vi "Create Zero Plane.vi"(7 "3D Waterfall Property":T1={"General Property"={"Plot Name"="", "Coordinate System"=enum."Cartesian", "Opacity"=0.0}, "Projection Property"={"Draw XY"=FALSE, "Draw YZ"=FALSE, "Draw XZ"=FALSE}, "Plot Property"={"Line Style"=enum."None", "Line Width"=0.0, "Color Ramp Cluster"={"Color Ramp Style"=enum."None", "Color Ramp Array"=[16711934, 393471, 57855, 4390754, 16449346, 16744722, 16711680], "Color Ramp Index"=[45, 91, 133, 175, 219, 255], "Interpolate?"=FALSE, "Logarithm?"=FALSE}, "Antialiasing"=FALSE}, "Waterfall Property"={"Waterfall Mode"=enum."Lines"}}, 8 "error in (no error)":errorcluster, 9 "Actual Transform In":T7, 10 "Plot Representation In":T4, 11 "Plot Object In":refnum<vi>) -> (0 "error out":errorcluster, 1 "Actual Transform Out":T7, 2 "Plot Representation Out":T4, 3 "Plot Object Out":refnum<vi>, 4 "Zero Plane Object Out":refnum<vi>)   [LabVIEW 2017, in "3D Waterfall.lvclass"]
uses:
  <vilib>/Math Plots/3D Math Plots/3D Waterfall/3D Waterfall/3D Waterfall.lvclass
  <vilib>/Math Plots/3D Math Plots/3D Plot/3D Plot/Typedef/Actual Transform.ctl
  <vilib>/Math Plots/3D Math Plots/3D Plot/3D Plot/Typedef/Range Clusters.ctl
  <vilib>/Math Plots/3D Math Plots/3D Plot/3D Plot/Typedef/Plot Representation.ctl
  <vilib>/Math Plots/3D Math Plots/3D Plot/3D Plot/Typedef/Mesh Data.ctl
  <vilib>/Math Plots/3D Math Plots/3D Waterfall/3D Waterfall/Typedef/3D Waterfall Property.ctl
  <vilib>/Math Plots/3D Math Plots/3D Plot/3D Plot/Typedef/Line Type.ctl
  <vilib>/Math Plots/3D Math Plots/3D Plot/3D Plot/Typedef/Color Ramp Cluster.ctl
  <vilib>/picture/3D Picture Control/NI_3D Picture Control.lvlib
  <vilib>/Math Plots/3D Math Plots/3D Plot/3D Plot/3D Plot.lvclass
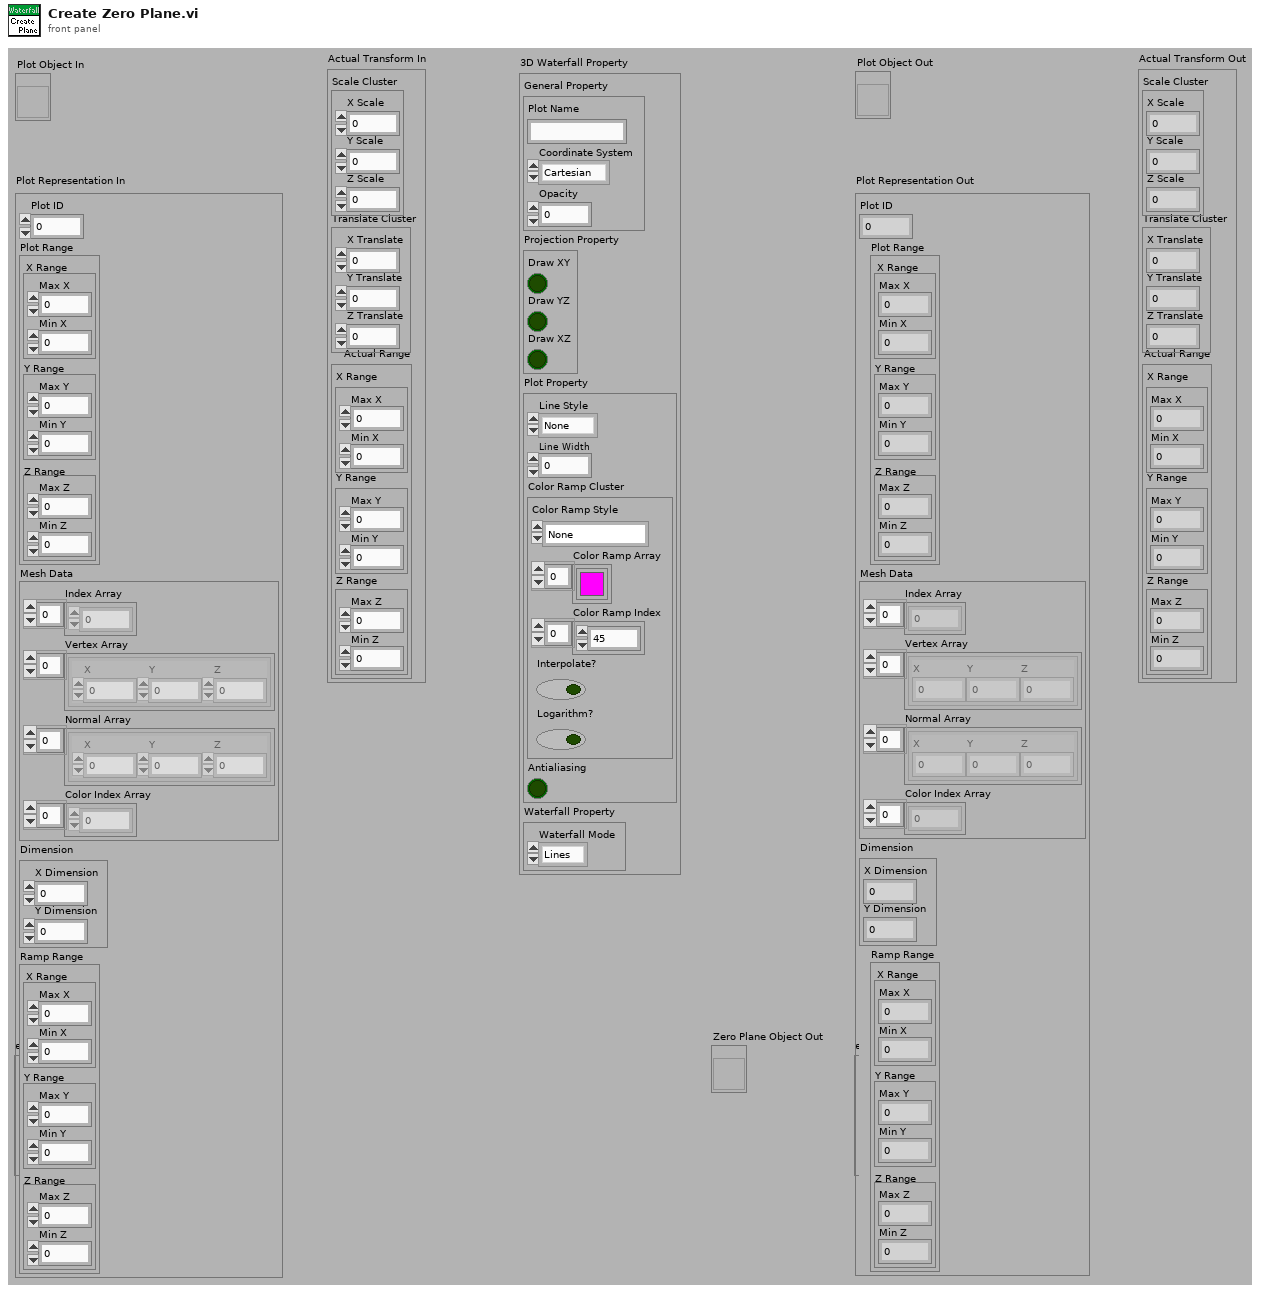
[diagram p1: front panel]
types:
  T1 = typedef "3D Waterfall.lvclass/3D Waterfall Property.ctl" = cluster{"General Property":cluster{"Plot Name":string, "Coordinate System":enum16{"Cartesian", "Cylindrical", "Spherical"}, "Opacity":sgl}, "Projection Property":cluster{"Draw XY":bool, "Draw YZ":bool, "Draw XZ":bool}, "Plot Property":cluster{"Line Style":T2, "Line Width":sgl, "Color Ramp Cluster":T3, "Antialiasing":bool}, "Waterfall Property":cluster{"Waterfall Mode":enum16{"Lines", "Slices"}}}
  T2 = typedef "3D Plot.lvclass/Line Type.ctl" = enum16{"None", "Solid", "Dash", "Dot", "Dash Dot"}
  T3 = typedef "3D Plot.lvclass/Color Ramp Cluster.ctl" = cluster{"Color Ramp Style":enum16{"None", "Shaded", "Color spectrum", "Grey scale", "Custom"}, "Color Ramp Array":u32[], "Color Ramp Index":i32[], "Interpolate?":bool, "Logarithm?":bool}
  T4 = typedef "3D Plot.lvclass/Plot Representation.ctl" = cluster{"Plot ID":i32, "Plot Range":T5, "Mesh Data":T6, "Dimension":cluster{"X Dimension":i32, "Y Dimension":i32}, "Ramp Range":T5}
  T5 = typedef "3D Plot.lvclass/Range Clusters.ctl" = cluster{"X Range":cluster{"Max X":sgl, "Min X":sgl}, "Y Range":cluster{"Max Y":sgl, "Min Y":sgl}, "Z Range":cluster{"Max Z":sgl, "Min Z":sgl}}
  T6 = typedef "3D Plot.lvclass/Mesh Data.ctl" = cluster{"Index Array":u32[], "Vertex Array":cluster{"X":sgl, "Y":sgl, "Z":sgl}[], "Normal Array":cluster{"X":sgl, "Y":sgl, "Z":sgl}[], "Color Index Array":i32[]}
  T7 = typedef "3D Plot.lvclass/Actual Transform.ctl" = cluster{"Scale Cluster":cluster{"X Scale":sgl, "Y Scale":sgl, "Z Scale":sgl}, "Translate Cluster":cluster{"X Translate":sgl, "Y Translate":sgl, "Z Translate":sgl}, "Actual Range":T5}
  T8 = enum16{"Overall", "Per Primitive", "Per Vertex", "Binding Off"}
  T9 = enum16{"Points", "Lines", "Line Strip", "Line Loop", "Triangles", "Triangle Strip", "Triangle Fan", "Quads", "Quad Strip", "Polygon"}
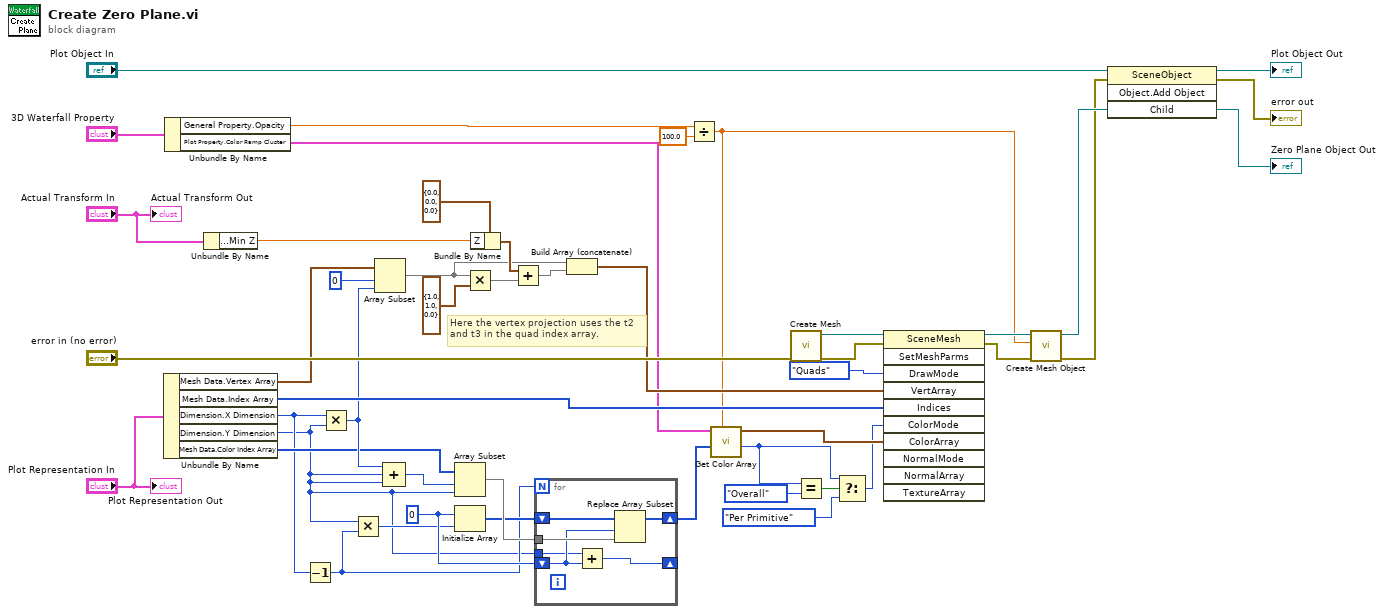
[diagram p0: block diagram]
diagram:
  w10 = 0 ("element")
  # "Here the vertex projection uses the t2\nand t3 in the quad index array."
  n1 = Unbundle By Name("Plot Representation In") -> ("Mesh Data.Vertex Array"=w29:cluster{"X":sgl, "Y":sgl, "Z":sgl}[], "Mesh Data.Index Array"=w35:u32[], "Dimension.X Dimension"=w13:i32, "Dimension.Y Dimension"=w6:i32, "Mesh Data.Color Index Array"=w15:i32[])
  n2 = Unbundle By Name("3D Waterfall Property") -> ("General Property.Opacity"=w40:sgl, "Plot Property.Color Ramp Cluster"=w19:T3)
  n3 = Unbundle By Name("Actual Transform In") -> ("Actual Range.Z Range.Min Z"=w31:sgl)
  n4 = Decrement(x=w13) -> (x-1=w9:i32)
  n5 = Multiply(x=w13, y=w6) -> (x*y=w16:i32)
  n6 = Multiply(x=w6, y=w9) -> (x*y=w8:i32)
  n7 = Array Subset(array=w29, index=0, length=w16) -> (w28:cluster{"X":sgl, "Y":sgl, "Z":sgl}[])
  n8 = Compound Arithmetic op=ADD(w16, w6, w6) -> (w14:i32)
  n9 = Array Subset(array=w15, index=w14, length=w6) -> (w12:i32[])
  n10 = Initialize Array(w10, w8) -> (w11:i32[])
  n11 = Multiply(x=w28, y=cluster{"X":sgl, "Y":sgl, "Z":sgl} {"X"=1.0, "Y"=1.0, "Z"=0.0} ("3D Point 2")) -> (x*y=w33:cluster{"X":sgl, "Y":sgl, "Z":sgl}[])
  n12 = Bundle By Name(cluster=cluster{"X":sgl, "Y":sgl, "Z":sgl} {"X"=0.0, "Y"=0.0, "Z"=0.0} ("3D Point 2"), "Z"=w31) -> (w32:cluster{"X":sgl, "Y":sgl, "Z":sgl})
  n13 = Add(x=w32, y=w33) -> (x+y=w30:cluster{"X":sgl, "Y":sgl, "Z":sgl}[])
  n14 = for {
    N: w9 -> [_]
    tunnel: w12 -> [w51]
    shift-right: [w53] -> w7
    shift-left: w11 -> [w52]
    shift-right: [w49] -> _
    shift-left: w10 -> [w50]
    tunnel: w6 -> [w48]
    n15 = Add(x=w48, y=w50) -> (x+y=w49:i32)
    n16 = Replace Array Subset(array=w52, new element=w51, index=w50) -> (w53:i32[])
  }
  n17 = Build Array (concatenate)(w28, w30) -> (w34:cluster{"X":sgl, "Y":sgl, "Z":sgl}[])
  n18 = Divide(x=w40, y=sgl 100.0) -> (x/y=w17:sgl)
  n19 = call <vilib>:"Get Color Array.vi"("Alpha"=w17, "Color Index Array"=w7, "Color Ramp Cluster"=w19) -> ("Color Binding Mode"=w3:T8, "Color Array"=w18:cluster{"R":sgl, "G":sgl, "B":sgl, "A":sgl}[])  [unwired: 4 in, 3 out]
  n20 = call <vilib>:"Create Mesh.vi"("error in (no error)"="error in (no error)") -> ("error out"=w38:errorcluster, "New Mesh Refnum"=w39:refnum<vi>)  [unwired: 9 out]
  n21 = Equal?(x=w3, y=T8."Overall") -> (x = y?=w4:bool)
  n22 = Select(t=w3, s=w4, f=T8."Per Primitive" ("Color Binding Mode")) -> (s? t:f=w1:T8)
  n23 = invoke class="SceneMesh" method="SetMeshParms"(reference=w39, error in=w38, "DrawMode"=T9."Quads" ("Draw Mode"), "VertArray"=w34, "Indices"=w35, "ColorMode"=w1, "ColorArray"=w18) -> (reference out=w26:refnum<vi>, error out=w27:errorcluster)  [unwired: 4 in, 9 out]
  n24 = call <vilib>:"Create Mesh Object.vi"("error in (no error)"=w27, "Alpha"=w17, "Mesh Object In"=w26) -> ("error out"=w24:errorcluster, "Object Ref Out"=w25:refnum<vi>)  [unwired: 1 in, 6 out]
  n25 = invoke class="SceneObject" method="Object.Add Object"(reference="Plot Object In", error in=w24, "Child"=w25) -> (reference out=→"Plot Object Out":refnum<vi>, error out=→"error out":errorcluster, "Child"=→"Zero Plane Object Out":refnum<vi>)  [unwired: 1 in, 1 out]
  "Actual Transform Out" <- "Actual Transform In"
  "Plot Representation Out" <- "Plot Representation In"
